vi "pcfs_initialize_log.vi"(8 "error in (no error)":errorcluster, 11 "pcfs in":refnum<class "pcfs.lvclass">) -> (0 "error out":errorcluster, 3 "pcfs out":refnum<class "pcfs.lvclass">)   [LabVIEW 2015, in "pcfs.lvclass"]
uses:
  pcfs.lvclass
  pcfs.lvclass/pcfs.ctl
  pcfs_log/pcfs_hdf5_log.lvclass
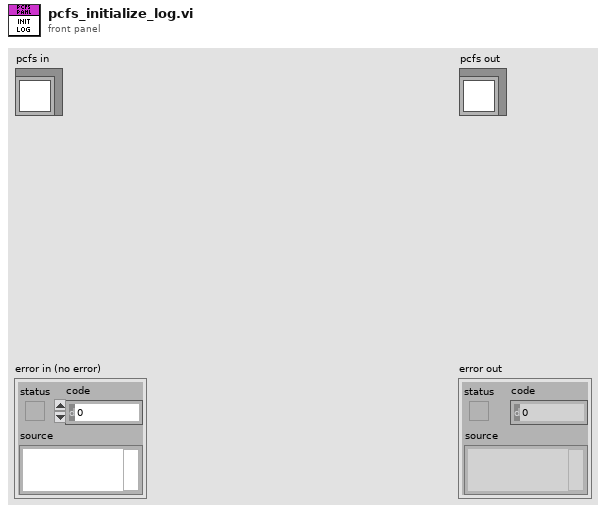
[diagram p1: front panel]
types:
  T1 = typedef "pcfs_settings.ctl" = cluster{"Center Pos. (mm)":dbl, "Increment (mm)":dbl, "Steps":dbl, "Dither Dist (nm)":dbl, "Dither Period (s)":dbl, "Cycles":dbl, "Record Type":T2, "Save Path":path, "Stage Number":enum16{"1", "2"}, "File Notes":string, "Mode":T3, "overwrite":bool, "custom_path":bool, "custom_positions":dbl[]}
  T2 = typedef "scan_record.ctl" = enum16{"hdf5", "legacy", "None"}
  T3 = typedef "hpanel_acq_modes.ctl" = u16
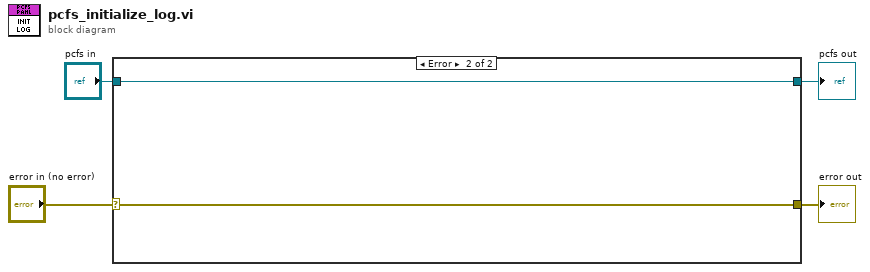
[diagram p0: block diagram]
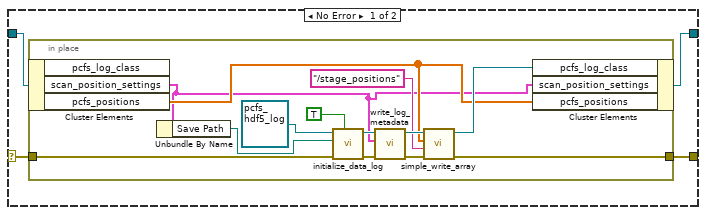
[diagram p2: hidden frame]
diagram:
  n1 = case shown="Error" "error in (no error)" {
    selector: "error in (no error)" -> [w6 w22]
    tunnel: [w5 w23] -> w2
    tunnel: "pcfs in" -> [w8 w23]
    tunnel: [w7 w22] -> w1
    frame No Error {
      n2 = in-place {
        in-place-border: [w14] -> w7
        in-place-border: w6 -> [w13]
        n3 = in-place-cluster #1(w8) -> ("scan_position_settings"=w10:T1, "pcfs_positions"=w11:dbl[])  [unwired: 1 out]
        n4 = Unbundle By Name(w10) -> ("Save Path"=w9:path)
        n5 = call-dynamic "initialize_data_log.vi"("Overwrite?"=TRUE, "error in (no error)"=w13, "Path"=w9, "pcfs_hdf5_log in"=refnum<class "pcfs_hdf5_log.lvclass"> refnum) -> ("error out"=w19:errorcluster, "pcfs_hdf5_log out"=w18:refnum<class "pcfs_hdf5_log.lvclass">)  [unwired: 6 in]
        n6 = call-dynamic "write_log_metadata.vi"("error in (no error)"=w19, "data"=w10, "pcfs_hdf5_log in"=w18) -> ("error out"=w16:errorcluster, "pcfs_hdf5_log out"=w17:refnum<class "pcfs_hdf5_log.lvclass">)  [unwired: 7 in]
        n7 = call-dynamic "simple_write_array.vi"("error in (no error)"=w16, "path"="/stage_positions", "Array"=w11, "pcfs_hdf5_log in"=w17) -> ("error out"=w14:errorcluster, "pcfs_hdf5_log out"=w15:refnum<class "pcfs_hdf5_log.lvclass">)  [unwired: 6 in]
        n8 = in-place-cluster #1("pcfs_log_class"=w15, "scan_position_settings"=w10, "pcfs_positions"=w11) -> (w5:refnum<class "pcfs.lvclass">)
      }
    }
    frame Error {
    }
  }
  "error out" <- w1
  "pcfs out" <- w2
